vi "INI Read write DBL 2D storage.vi"(6 "Values to write":dbl[][](array[numeric]), 7 "Read/Write mode":T1, 8 "error in":errorcluster, 9 "Defaults":dbl[][](array[numeric]), 10 "key":string, 11 "section":string) -> (0 "error out":errorcluster, 2 "Values":dbl[][](array[numeric]))   [LabVIEW 2010]
doc: "This module is used to store and retrieve information from the .ini file. On first call, it reads from the file on disk and stores the information in memory."
uses:
  Read write mode.ctl
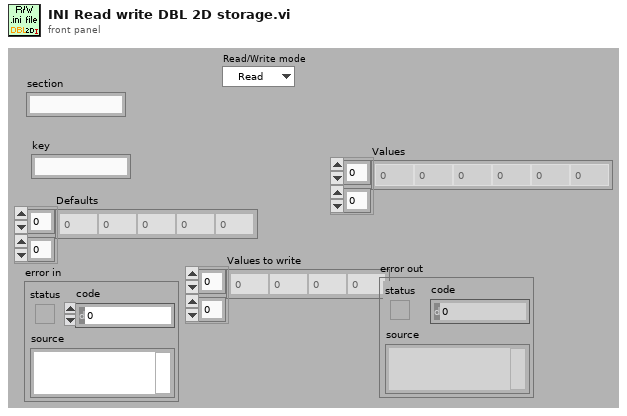
[diagram p1: front panel]
types:
  T1 = typedef "Read write mode.ctl" = enum16{"Read", "Write"}
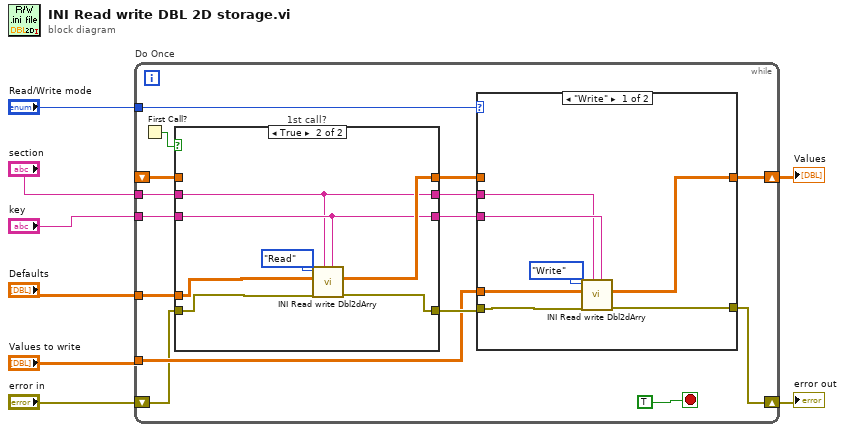
[diagram p0: block diagram]
diagram:
  n1 = while "Do Once" {
    tunnel: "section" -> [w21]
    tunnel: "Read/Write mode" -> [w20]
    tunnel: "Values to write" -> [w13]
    tunnel: "key" -> [w15]
    shift-right: [w12] -> w7
    shift-left: _ -> [w14]
    tunnel: "Defaults" -> [w9]
    shift-right: [w10] -> w3
    shift-left: "error in" -> [w11]
    stop <- TRUE stop-if-true
    n2 = First Call?() -> (First Call?: T/F=w22:bool)
    n3 = case "1st call?" shown="True" w22 {
      tunnel: w21 -> [w36 w39]
      tunnel: w15 -> [w35 w42]
      tunnel: [w34 w43] -> w16
      tunnel: [w33 w38] -> w19
      tunnel: [w36 w39] -> w18
      tunnel: [w35 w42] -> w17
      tunnel: w14 -> [w34 _]
      tunnel: w11 -> [w33 w41]
      tunnel: w9 -> [_ w40]
      frame False {
      }
      frame True {
        n4 = call "INI Read write Dbl2dArry.vi"("key"=w42, "section"=w39, "error in"=w41, "dbl array in"=w40, "Read|Write"=Read_write_mode."Read") -> ("error out"=w38:errorcluster, "dbl array out"=w43:dbl[][])  [unwired: 5 in]
      }
    }
    n5 = case "1st call?" shown="\"Write\"" w20 {
      tunnel: w19 -> [w30 w31]
      tunnel: w18 -> [w26 _]
      tunnel: w17 -> [w29 _]
      tunnel: [w28 w32] -> w12
      tunnel: [w25 w31] -> w10
      tunnel: w16 -> [_ w32]
      tunnel: w13 -> [w27 _]
      frame "Write" {
        n6 = call "INI Read write Dbl2dArry.vi"("key"=w29, "section"=w26, "error in"=w30, "dbl array in"=w27, "Read|Write"=Read_write_mode."Write") -> ("error out"=w25:errorcluster, "dbl array out"=w28:dbl[][])  [unwired: 5 in]
      }
      frame "Read" {
      }
    }
  }
  "Values" <- w7
  "error out" <- w3
